vi "Register Memory or Image Event.vi"   [LabVIEW 2012]
doc: "Registers a memory or image user event using a Boolean Labview User Event. Once memory or image has been registered with a Labview User Event, it can be read and written to asynchronously (non-blocking) to allow other tasks to be performed by the program including user inputs to the front panel.\n\nThis is useful when copying very large datasets to the device."
uses:
  OpenCLV x64.lvlib
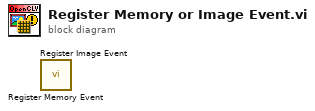
[diagram p0: block diagram]
diagram:
  n1 = call "Register Memory Event.vi"() -> ()  [unwired: 9 in, 3 out]
  n2 = call "Register Image Event.vi"() -> ()  [unwired: 9 in, 3 out]
